vi "SV Multitone Gain and Phase.vi"   [LabVIEW 2017, in "SoundVib_Multitone.lvlib"]
doc: "Use this VI to measure the gain and phase versus frequency. Wire data to <B>scaled signal [EU]</B> to determine the polymorphic instance to use or manually select the instance."
uses:
  <vilib>/addons/Sound and Vibration/svt_Multitone Distortion/SoundVib_Multitone.lvlib
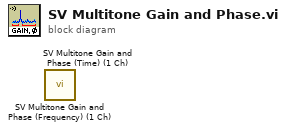
[diagram p0: block diagram]
diagram:
  n1 = call <vilib>:"SV Multitone Gain and Phase (Frequency) (1 Ch).vi"() -> ()  [unwired: 13 in, 7 out]
  n2 = call <vilib>:"SV Multitone Gain and Phase (Time) (1 Ch).vi"() -> ()  [unwired: 13 in, 7 out]
